vi "TCP_open_write_read_close.vi"(4 "timeout ms (25000)":i32, 5 "bytes to read":i32, 6 "mode (standard)":T1(ring), 7 "write string":string, 8 "error in":errorcluster, 9 "local port (0)":u16, 10 "remote port or service name":u16, 11 "address":string) -> (0 "error out":errorcluster, 3 "read string":string)   [LabVIEW 2020]
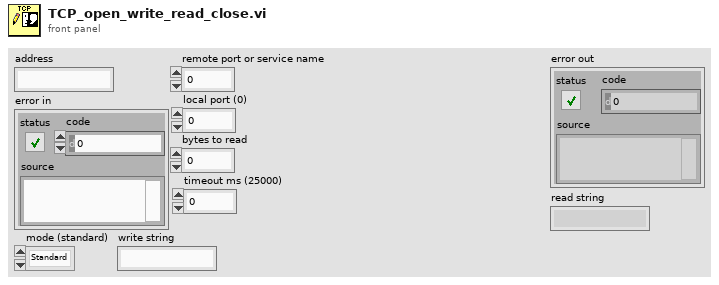
[diagram p1: front panel]
types:
  T1 = enum16{"Standard", "Buffered", "CRLF", "Immediate"}
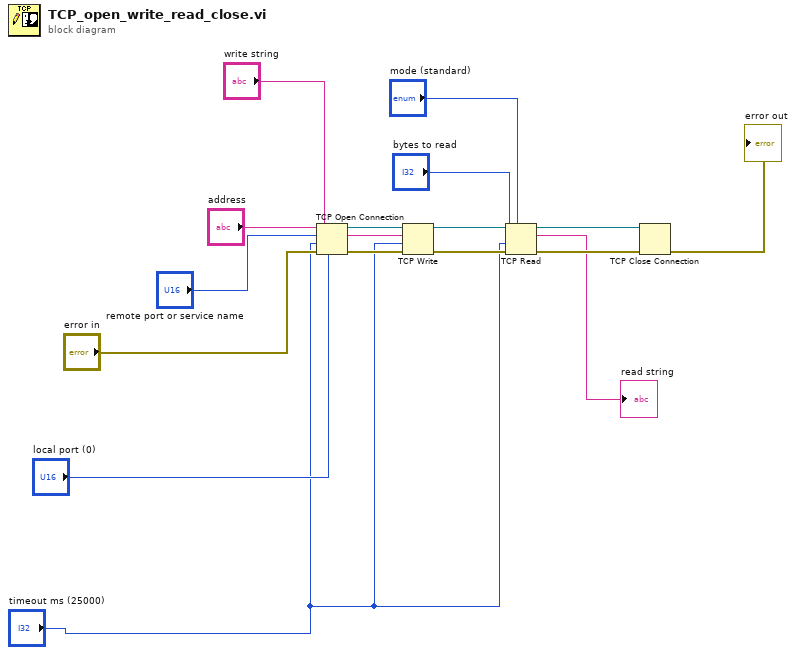
[diagram p0: block diagram]
diagram:
  n1 = TCP Open Connection(address="address", remote port or service name="remote port or service name", timeout ms (60000)="timeout ms (25000)", local port="local port (0)", error in (no error)="error in") -> (connection ID=w14:refnum<k5>, error out=w13:errorcluster)
  n2 = TCP Write(connection ID=w14, data in="write string", error in (no error)=w13, 9:"timeout ms (25000)") -> (connection ID out=w12:refnum<k5>, error out=w11:errorcluster)  [unwired: 1 out]
  n3 = TCP Read(connection ID=w12, bytes to read="bytes to read", error in (no error)=w11, 7:"mode (standard)", 9:"timeout ms (25000)") -> (connection ID out=w10:refnum<k5>, data out=→"read string":string, error out=w9:errorcluster)
  n4 = TCP Close Connection(connection ID=w10, error in (no error)=w9) -> (error out=→"error out":errorcluster)  [unwired: 1 in, 1 out]
